vi "Linear.vi"(5 "distances":dbl[](array[numeric]), 6 "return immediately":bool, 7 "speed":dbl, 8 "error in (no error)":errorcluster, 9 "taskId":i32(ring) items=["TLibrary", "T01", "T02", "T03", "T04", "T05", "T06", "T07", "T08", "T09", "T10", "T11", "T12", "T13", "T14", "T15", "T16", "T17", "T18", "T19", "T20", "T21", "T22", "T23", "T24", "T25", "T26", "T27", "T28", "T29", "T30", "T31"], 10 "axis names":string[](array[string]), 11 "controller in":refnum<k24>) -> (0 "error out":errorcluster, 3 "controller out":refnum<k24>)   [LabVIEW 2011]
uses:
  C:/Users/Admin/Desktop/Gantry Code Transfer/source/Code Transfer/Aerotech.A3200.dll
  Aerotech.A3200.dll
  C:/Users/Admin/Desktop/Gantry Code Transfer/source/Code Transfer/Aerotech.A3200.LabVIEW.dll
  Aerotech.A3200.LabVIEW.dll
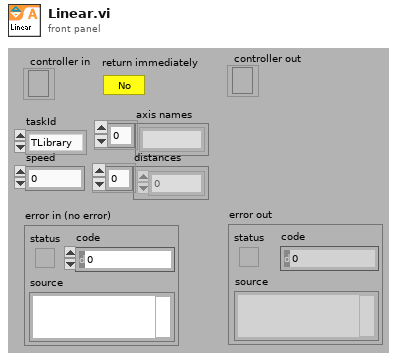
[diagram p1: front panel]
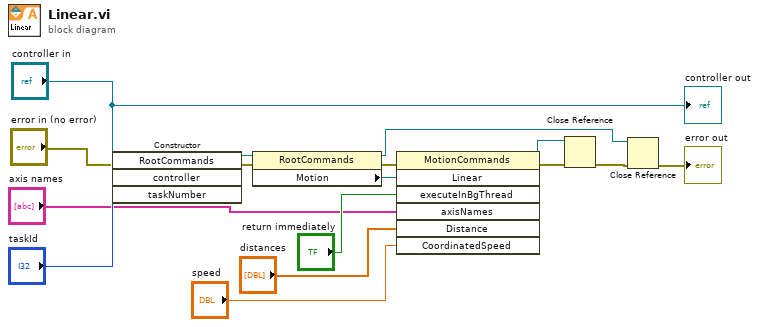
[diagram p0: block diagram]
diagram:
  n1 = constructor class="RootCommands"(error in="error in (no error)", "controller"="controller in", "taskNumber"="taskId") -> (reference out=w8:refnum<k24>, error out=w9:errorcluster)  [unwired: 2 in, 3 out]
  n2 = property class="RootCommands"(reference=w8, error in=w9) -> (reference out=w5:refnum<k24>, error out=w7:errorcluster, "Motion"=w6:refnum<k24>)
  n3 = invoke class="MotionCommands" method="Linear"(reference=w6, error in=w7, "executeInBgThread"="return immediately", "axisNames"="axis names", "Distance"="distances", "CoordinatedSpeed"="speed") -> (reference out=w11:refnum<k24>, error out=w10:errorcluster)  [unwired: 1 in, 5 out]
  n4 = Close Reference(reference=w11, error in (no error)=w10) -> (error out=w12:errorcluster)
  n5 = Close Reference(reference=w5, error in (no error)=w12) -> (error out=→"error out":errorcluster)
  "controller out" <- "controller in"
